vi "SECoP_dataCreateString.vi"(6 "value":string, 8 "error in (no error)":errorcluster, 11 "DLL path (in)":T2) -> (0 "error out":errorcluster, 2 "SECoP_dataPtr (out)":T1 {"ptr64" format="%.0x"; "ptr32" format="%.0x"}, 3 "DLL path (out)":T2)   [LabVIEW 2023, in "SECoP.lvlib"]
doc: "Call <b>\"SECoP_dataCreateString.vi\"</b> to create a simple string (text) data type and set value. Free resources after use with <b>\"SECoP_dataDestroy.vi\"</b>.\n\n<b>DLL path</b> input and output of cluster from \"SECoP-Initialize.vi\"\n<b>value</b> new value\n<b>SECoP_dataPtr</b> created data"
uses:
  SECoP.lvlib
  SECoP-libraries.ctl
  SECoP-data.ctl
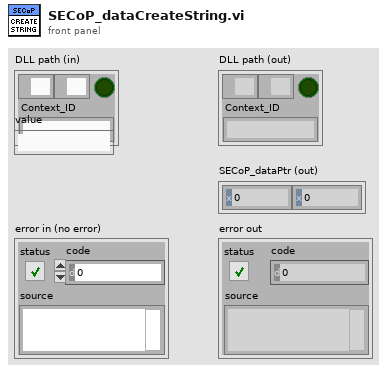
[diagram p1: front panel]
types:
  T1 = typedef "SECoP.lvlib/SECoP-data.ctl" = cluster{"ptr32":u32, "ptr64":u64}
  T2 = typedef "SECoP.lvlib/SECoP-libraries.ctl" = cluster{"serverDLL":path, "variantDLL":path, "cleanup_mode":bool, "Context_ID":string}
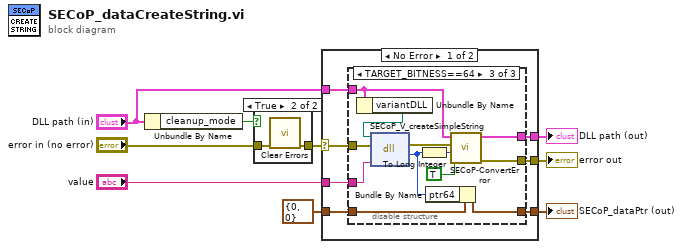
[diagram p0: block diagram]
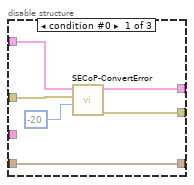
[diagram p3: hidden frame]
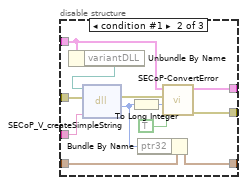
[diagram p4: hidden frame]
diagram:
  n1 = Unbundle By Name("DLL path (in)") -> ("cleanup_mode"=w7:bool)
  n2 = case shown="True" w7 {
    tunnel: "error in (no error)" -> [w10 w12]
    tunnel: [w10 w11] -> w5
    frame False {
    }
    frame True {
      n3 = call <vilib>:"Clear Errors.vi"("error in (no error)"=w12) -> ("error out"=w11:errorcluster)  [unwired: 5 in, 1 out]
    }
  }
  n4 = case shown="No Error" w5 {
    selector: w5 -> [w19 w51]
    tunnel: "DLL path (in)" -> [w18 w52]
    tunnel: [w16 w52] -> w9
    tunnel: [w17 w51] -> w8
    tunnel: [w14 w50] -> w4
    tunnel: T1 {"ptr32"=0, "ptr64"=0} ("SECoP_dataPtr (out)") -> [w15 w50]
    tunnel: "value" -> [w13 _]
    frame No Error {
      n5 = disable-structure shown="TARGET_BITNESS==64" {
        disable-tunnel: w19 -> [w25 w37 w49]
        disable-tunnel: w18 -> [w24 w26 w39]
        disable-tunnel: [w22 w33 w45] -> w17
        disable-tunnel: [w23 w32 w44] -> w16
        disable-tunnel: w15 -> [w20 w35 w47]
        disable-tunnel: [w20 w36 w48] -> w14
        disable-tunnel: w13 -> [_ w28 w40]
        frame condition #0 {
          n6 = call "SECoP-ConvertError.vi"("return code"=-20, "error in (no error)"=w25, "DLL path (in)"=w24) -> ("error out"=w22:errorcluster, "DLL path (out)"=w23:T2)  [unwired: 7 in]
        }
        frame condition #1 {
          n7 = Unbundle By Name(w26) -> ("variantDLL"=w27:path)
          n8 = dll-call lib="Z:/Praktische_Aufgaben/SECoP-LabVIEW2015/32bit/SECoP32.dll" fn="SECoP_V_createSimpleString"(path in=w27, error in=w37, "szValue"=w28) -> (error out=w34:errorcluster, "return type"=w31:u32)  [unwired: 2 in, 1 out]
          n9 = To Long Integer(number=w31) -> (32bit integer=w29:i32)
          n10 = Bundle By Name(cluster=w35, "ptr32"=w31) -> (w36:T1)
          n11 = call "SECoP-ConvertError.vi"("return is boolean"=TRUE, "return code"=w29, "error in (no error)"=w34, "DLL path (in)"=w26) -> ("error out"=w33:errorcluster, "DLL path (out)"=w32:T2)  [unwired: 6 in]
        }
        frame condition #2 (active) {
          n12 = Unbundle By Name(w39) -> ("variantDLL"=w38:path)
          n13 = dll-call lib="Z:/Praktische_Aufgaben/SECoP-LabVIEW2015/32bit/SECoP32.dll" fn="SECoP_V_createSimpleString"(path in=w38, error in=w49, "szValue"=w40) -> (error out=w46:errorcluster, "return type"=w43:u64)  [unwired: 2 in, 1 out]
          n14 = To Long Integer(number=w43) -> (32bit integer=w41:i32)
          n15 = Bundle By Name(cluster=w47, "ptr64"=w43) -> (w48:T1)
          n16 = call "SECoP-ConvertError.vi"("return is boolean"=TRUE, "return code"=w41, "error in (no error)"=w46, "DLL path (in)"=w39) -> ("error out"=w45:errorcluster, "DLL path (out)"=w44:T2)  [unwired: 6 in]
        }
      }
    }
    frame Error {
    }
  }
  "DLL path (out)" <- w9
  "error out" <- w8
  "SECoP_dataPtr (out)" <- w4
